vi "RunMeas.vi"(8 "error in (no error)":errorcluster, 11 "NHRDCModel in":refnum<class "NHRDCPowerModel.lvclass">) -> (0 "error out":errorcluster, 2 "variant":variant, 3 "NHRDCModel out":refnum<class "NHRDCPowerModel.lvclass">)   [LabVIEW 2018, in "AcPwrPlugins.lvlib" / "NHRDCPowerModel.lvclass"]
doc: "This VI initiates and takes measurements from the instrument(s)."
uses:
  NHRDCPowerModel.lvclass
  AcPwrShared/clMeasurmentData.ctl
  AcPwrShared/clEventType.ctl
  AcPwrBaseClass/AcPwrBase.lvclass
  AcPwrShared/AcPwrShared.lvlib
panel:
  in  "Measurement Type":enum16{"Voltage", "Current", "Power"}(ring)
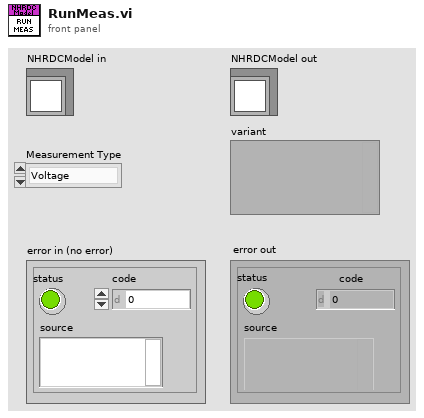
[diagram p1: front panel]
types:
  T1 = typedef "AcPwrShared.lvlib/clMeasurmentData.ctl" = cluster{"MeasName":string, "XML Data":string, "WaveformData":waveform(dbl)[]}
  T2 = typedef "AcPwrShared.lvlib/clEventType.ctl" = cluster{"ModuleID":i32, "Data":variant}
  T3 = cluster{"Handle":string, "Name":string, "Enabled":bool, "Measurement Value":sgl, "Measurement Type":enum16{"Power", "Current", "Voltage"}}
  T4 = typedef "AcPwrPlugins.lvlib/NHRDCPower.lvclass/Measurements.ctl" = cluster{"Handle":string, "Name":string, "Enabled":bool, "Measurement Value":sgl, "Measurement Type":enum16{"Power", "Current", "Voltage"}}[]
  T5 = typedef "AcPwrPlugins.lvlib/NHRDCPower.lvclass/Device(s)Settings.ctl" = cluster{"MeasName":string, "Modules":T6}
  T6 = typedef "AcPwrPlugins.lvlib/NHRDCPower.lvclass/Modules.ctl" = cluster{"Handle":string, "Name":string, "id query (Yes)":bool, "reset device (Yes)":bool, "Connected":bool, "Initial Battery Detect Voltage (0)":dbl, "SafetySettings":cluster{"SetWatchDog?":bool, "Voltage (V)":dbl, "Current (A)":dbl, "Power (W)":dbl, "Voltage Delay (s)":dbl, "Current Delay (s)":dbl, "Power Delay (s)":dbl}, "Options String":string, "Aperture Time (s)":dbl, "operating state (Off)":i32, "OutputSettings":cluster{"Voltage (V)":dbl, "Current (A)":dbl, "Resistance (Ohms)":dbl, "Power (W)":dbl, "Enable Voltage":bool, "Enable Current":bool, "Enable Resistance":bool, "Enable Power":bool, "Macro After Step Delay  (s)":dbl, "Wait Value (V, A, W)":dbl, "Enable Wait":bool, "Wait on Value":i32}, "SlewRate":cluster{"Set Voltage Rate V/S":dbl, "Set Current Rate A/S":dbl, "Set Resistance Rate R/S":dbl, "Set Power Rate W/S":dbl}, "Macro":cluster{"Save Macro?":bool, "Load Macro From File?":bool, "Run Macro Continuously?":bool, "Use Macros?":bool, "Load Macro File Path":path, "Save Macro File Path":string}, "Regulation Gain (1=100%)":dbl, "UpdatingOntheFly":bool}[]
  T7 = typedef "AcPwrPlugins.lvlib/NHRDCPowerModel.lvclass/NHRDC_Model2ICDAS.ctl" = cluster{"data_id":i32, "voltage":dbl, "current":dbl, "power":dbl, "meas_timestamp":timestamp, "write_timestamp":timestamp, "read_by_icdas":bool, "read_timestamp":timestamp}
  T8 = typedef "AcPwrShared.lvlib/AcPwrBroadcastEvents.ctl" = cluster{"DidInit":refnum<user-event>, "StatusUpdate":refnum<user-event>, "ErrorReport":refnum<user-event>, "DidStop":refnum<user-event>, "PathToINI":refnum<user-event>, "Measurements":refnum<user-event>, "LoadConfigFile":refnum<user-event>, "GetSettings":refnum<user-event>, "SetSettings":refnum<user-event>, "GetType&ID":refnum<user-event>, "GotSettings":refnum<user-event>, "GotSettingsLV":refnum<user-event>, "ParameterSet":refnum<user-event>}
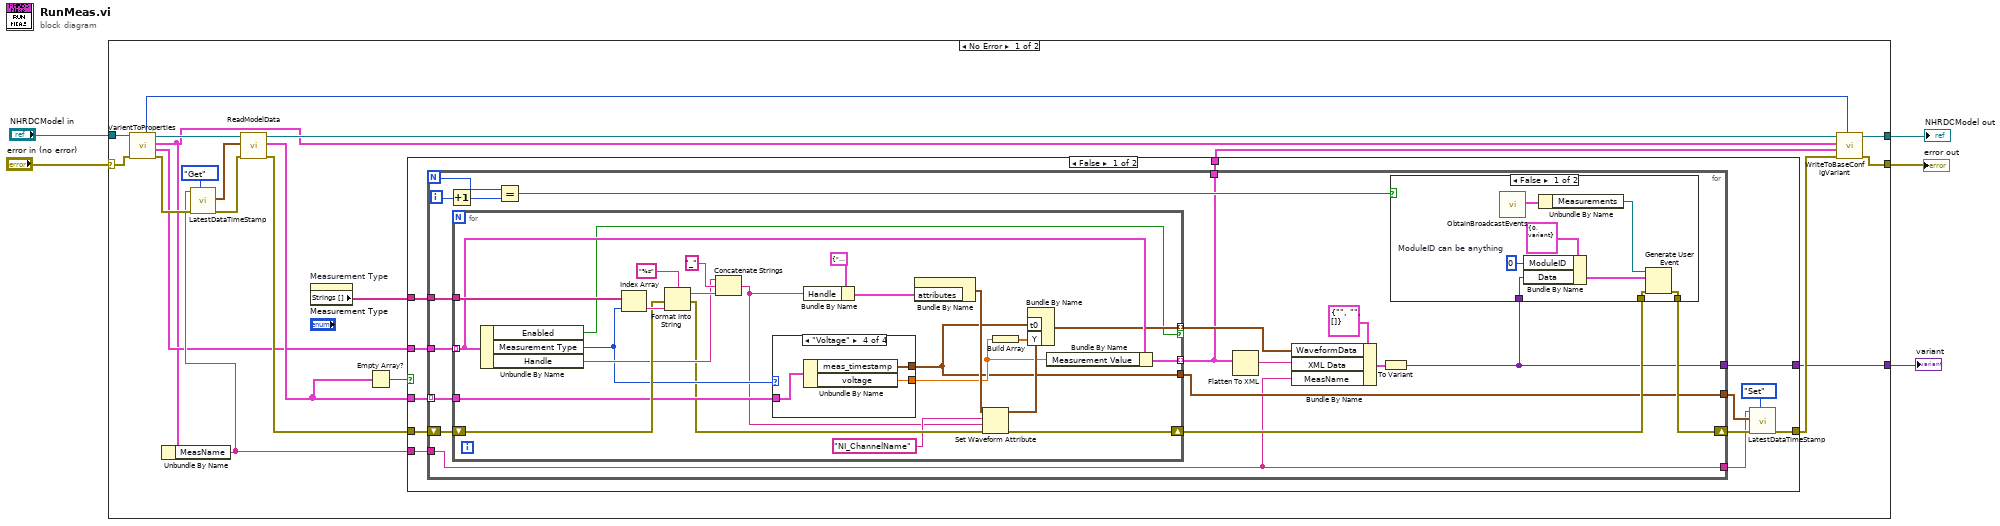
[diagram p0: block diagram]
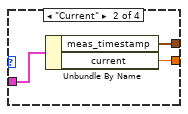
[diagram p4: hidden frame]
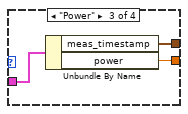
[diagram p5: hidden frame]
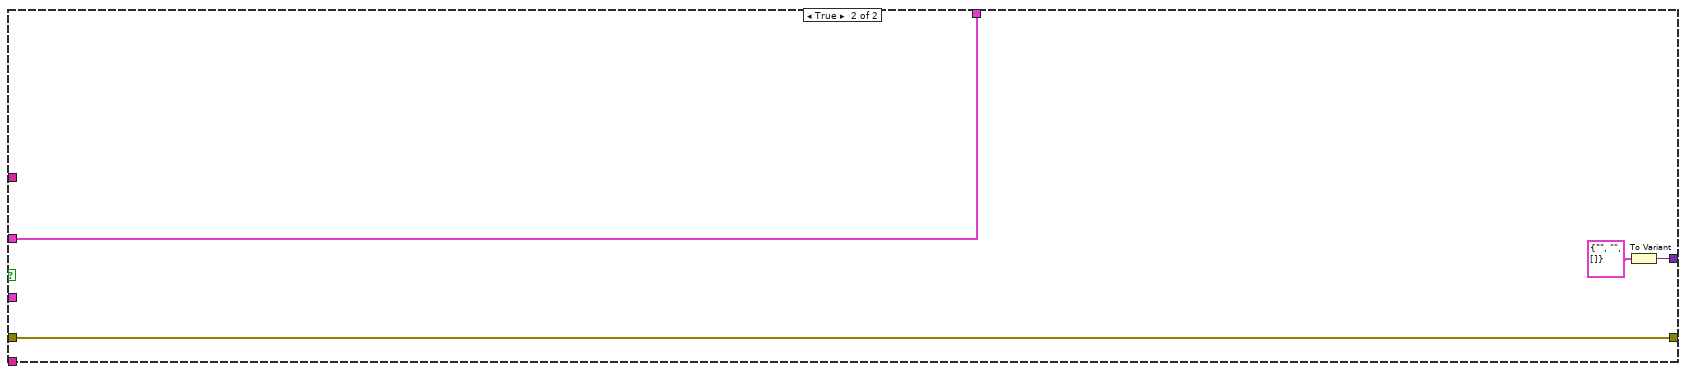
[diagram p6: hidden frame]
diagram:
  n1 = case shown="No Error" "error in (no error)" {
    selector: "error in (no error)" -> [w25 w104]
    tunnel: "NHRDCModel in" -> [w26 w103]
    tunnel: [w18 w104] -> w3
    tunnel: [w19 w103] -> w2
    tunnel: [w7 _] -> w1
    frame No Error {
      n2 = call "VarientToProperties.vi"("error in (no error)"=w25, "AcPwrPlugins.lvlib:NHRDCModel.lvclass"=w26) -> ("error out"=w22:errorcluster, "Measurements"=w13:T4, "Device(s)Settings"=w9:T5, "AcPwrPlugins.lvlib:NHRDCModel.lvclass"=w23:refnum<class "NHRDCPowerModel.lvclass">, "Measurement Refresh Time (ms)"=w6:u32)  [unwired: 4 in, 1 out]
      n3 = Unbundle By Name(w9) -> ("MeasName"=w14:string)
      n4 = call "LatestDataTimeStamp.vi"("Action"=enum16{"Set", "Get"}."Get", "error in (no error)"=w22, "Plugin Name"=w14) -> ("error IO"=w21:errorcluster, "Latest Data Timestamp"=w20:timestamp)  [unwired: 6 in, 1 out]
      n5 = call "ReadModelData.vi"("error in (no error)"=w21, "meas_timestamp in"=w20, "NHRDCModel in"=w23) -> ("error out"=w15:errorcluster, "Model2ICDAS Array"=w17:T7[], "NHRDCModel out"=w10:refnum<class "NHRDCPowerModel.lvclass">)  [unwired: 6 in]
      n6 = property on="Measurement Type" class="Enum (strict)"() -> ("Strings []"=w12:string[])  [unwired: 2 in, 2 out]
      n7 = Empty Array?(array=w17) -> (empty?=w16:bool)
      n8 = case shown="False" w16 {
        tunnel: w17 -> [w38 _]
        tunnel: w15 -> [w35 w99]
        tunnel: w14 -> [w34 _]
        tunnel: w13 -> [w37 w100]
        tunnel: w12 -> [w36 _]
        tunnel: [w29 w102] -> w7
        tunnel: [w28 w99] -> w8
        tunnel: [w27 w100] -> w11
        frame False {
          n9 = for {
            N -> [w53]
            tunnel: w38 -> [w55] mode=indexing
            tunnel: w37 -> [w56]
            tunnel: w36 -> [w51]
            shift-right: [w43] -> w32
            shift-left: w35 -> [w50]
            tunnel: w34 -> [w41]
            tunnel: [w42] -> w31
            tunnel: [w41] -> w30
            tunnel: [w40] -> w29
            tunnel: [w39] -> w27
            i -> [w54]
            n10 = Increment(x=w54) -> (x+1=w52:i32)
            n11 = for {
              tunnel: w56 -> [w73] mode=indexing
              tunnel: w55 -> [w81]
              tunnel: w51 -> [w89]
              shift-right: [w67] -> w44
              shift-left: w50 -> [w86]
              tunnel: [w71] -> w47 mode=indexing if=w69
              tunnel: [w70] -> w39 mode=indexing
              tunnel: [w68] -> w42
              n12 = Unbundle By Name(w73) -> ("Enabled"=w69:bool, "Measurement Type"=w80:enum16{"Power", "Current", "Voltage"}, "Handle"=w83:string)
              n13 = Index Array(array=w89, index=w80) -> (element=w87:string)
              n14 = Format Into String(format string="%s", error in=w86, w87) -> (resulting string=w85:string, error out=w79:errorcluster)  [unwired: 1 in]
              n15 = Concatenate Strings(w83, "_" ("string"), w85) -> (w77:string)
              n16 = case shown="\"Voltage\"" w80 {
                tunnel: w81 -> [_ w92 w95 w98]
                tunnel: [_ w91 w94 w97] -> w68
                tunnel: [_ w90 w93 w96] -> w72
                frame Default {
                }
                frame "Current" {
                  n17 = Unbundle By Name(w92) -> ("meas_timestamp"=w91:timestamp, "current"=w90:dbl)
                }
                frame "Power" {
                  n18 = Unbundle By Name(w95) -> ("meas_timestamp"=w94:timestamp, "power"=w93:dbl)
                }
                frame "Voltage" {
                  n19 = Unbundle By Name(w98) -> ("meas_timestamp"=w97:timestamp, "voltage"=w96:dbl)
                }
              }
              n20 = Bundle By Name(cluster=T3 {"Handle"="", "Name"="", "Enabled"=FALSE, "Measurement Value"=0.0, "Measurement Type"=enum."Power"} ("Measurement"), "Handle"=w77) -> (w82:T3)
              n21 = Bundle By Name("attributes"=w82) -> (w76:waveform(dbl))  [unwired: 1 in]
              n22 = Set Waveform Attribute(4:w79, 5:w77, 6:"NI_ChannelName" ("name"), 7:w76) -> (0:w67:errorcluster, 3:w75:waveform(dbl))  [unwired: 1 out]
              n23 = Build Array(w72) -> (w74:dbl[])
              n24 = Bundle By Name(cluster=w75, "t0"=w68, "Y"=w74) -> (w71:waveform(dbl))
              n25 = Bundle By Name(cluster=w73, "Measurement Value"=w72) -> (w70:T3)
            }
            n26 = Equal?(x=w53, y=w52) -> (x = y?=w45:bool)
            n27 = Flatten To XML(anything=w39) -> (xml string=w48:string)
            n28 = Bundle By Name(cluster=T1 {"MeasName"="", "XML Data"="", "WaveformData"=[]} ("MeasurmentDataCluster"), "WaveformData"=w47, "XML Data"=w48, "MeasName"=w41) -> (w46:T1)
            n29 = To Variant(anything=w46) -> (Variant=w40:variant)
            n30 = case shown="False" w45 {
              tunnel: w40 -> [w59 _]
              tunnel: w44 -> [w58 w65]
              tunnel: [w57 w65] -> w43
              frame False {
                w60 = 0  # ModuleID can be anything
                n31 = call "ObtainBroadcastEvents.vi"() -> ("AcPwrEvents"=w62:T8)  [unwired: 10 in, 1 out]
                n32 = Bundle By Name(cluster=T2 {"ModuleID"=0, "Data"=variant} ("clEventType"), "ModuleID"=w60, "Data"=w59) -> (w63:T2)
                n33 = Unbundle By Name(w62) -> ("Measurements"=w61:refnum<user-event>)
                n34 = Generate User Event(user event=w61, event data cluster=w63, error in=w58) -> (error out=w57:errorcluster)  [unwired: 1 in, 1 out]
              }
              frame True {
                # "Don't broadcast results for the last DB Record. The module should broadcast it after this VI is done."
              }
            }
          }
          n35 = call "LatestDataTimeStamp.vi"("Action"=enum16{"Set", "Get"}."Set", "error in (no error)"=w32, "TimeStamp"=w31, "Plugin Name"=w30) -> ("error IO"=w28:errorcluster)  [unwired: 5 in, 2 out]
        }
        frame True {
          n36 = To Variant(anything=T1 {"MeasName"="", "XML Data"="", "WaveformData"=[]} ("MeasurmentDataCluster")) -> (Variant=w102:variant)
        }
      }
      n37 = call-dynamic "WriteToBaseConfigVariant.vi"("Measurement Refresh Time (ms)"=w6, "error in (no error)"=w8, "Meas"=w11, "Config"=w9, "NHRDCModel in"=w10) -> ("error out"=w18:errorcluster, "NHRDCModel out"=w19:refnum<class "NHRDCPowerModel.lvclass">)  [unwired: 5 in]
    }
    frame Error {
    }
  }
  "NHRDCModel out" <- w2
  "error out" <- w3
  "variant" <- w1
